vi "stop async modules.vi"(7 "Variant":variant, 8 "error in":errorcluster, 11 "Engine Data Out in":T1={"timed loop timer source"={"Processor"=0, "Priority"=0, "timing source dt"=0, "timer source"=refnum}, "control loop data"={"engine tag bus"={"Double"=[], "Single"=[], "I64"=[], "I32"=[], "I16"=[], "I8"=[], "U64"=[], "U32"=[], "U16"=[], "U8"=[], "Boolean"=[], "String"=[], "Array of Double"=[], "Array of Single"=[], "Array of I64"=[], "Array of I32"=[], "Array of I16"=[], "Array of I8"=[], "Array of U64"=[], "Array of U32"=[], "Array of U16"=[], "Array of U8"=[], "Array of Boolean"=[], "Array of String"=[]}, "engine schedule"={"module run flags"=[], "decimation schedule"={"decimations"=[], "offsets"=[]}}, "module information"=[]}, "status reporting"={"late? index (bool)"=0, "late count index (U32)"=0, "dt (ns) index (U64)"=0, "execution time (ns) index (U64)"=-1}}) -> (0 "error out":errorcluster, 3 "Engine Data Out out":T1={"timed loop timer source"={"Processor"=0, "Priority"=0, "timing source dt"=0, "timer source"=refnum}, "control loop data"={"engine tag bus"={"Double"=[], "Single"=[], "I64"=[], "I32"=[], "I16"=[], "I8"=[], "U64"=[], "U32"=[], "U16"=[], "U8"=[], "Boolean"=[], "String"=[], "Array of Double"=[], "Array of Single"=[], "Array of I64"=[], "Array of I32"=[], "Array of I16"=[], "Array of I8"=[], "Array of U64"=[], "Array of U32"=[], "Array of U16"=[], "Array of U8"=[], "Array of Boolean"=[], "Array of String"=[]}, "engine schedule"={"module run flags"=[], "decimation schedule"={"decimations"=[], "offsets"=[]}}, "module information"=[]}, "status reporting"={"late? index (bool)"=0, "late count index (U32)"=0, "dt (ns) index (U64)"=0, "execution time (ns) index (U64)"=-1}})   [LabVIEW 2013, in "main engine.lvlib"]
doc: "Requests that all asynchronous modules abort as quickly as possible. When the modules return we swap their data back into the main cluster so they can pretend they are synchronous modules for future operations."
uses:
  main engine.lvlib
  Engine Data.ctl
  <vilib>/NI/Module Timing Source/timing source/TBM timing source.lvclass
  timed loop timing sources.ctl
  control loop data.ctl
  <vilib>/NI/Tag Bus/table/data table.ctl
  engine run schedule.ctl
  engine decimation schedule.ctl
  full module data.ctl
  <vilib>/NI/Tag Bus Module Framework/runtime/TBM module execution interface.lvclass
  module run state.ctl
  async executor/asynchronous executor reference.ctl
  async executor/async message to executor.ctl
  Runtime/async command notification.ctl
  Runtime/async error info.ctl
  <vilib>/NI/Tag Bus Module Framework/runtime/error classification.ctl
  <vilib>/NI/Tag Bus Module Framework/module configuration/TBM module configuration.lvclass
  module method data.ctl
  <vilib>/NI/Tag Bus/table/transfer specification.ctl
  <vilib>/NI/Tag Bus/tag/Data Type.ctl
  fault handling spec.ctl
  Configuration/Error Actions.ctl
  status reporting data.ctl
  <vilib>/NI/Tag Bus/table/data table.lvlib
  <vilib>/NI/Tag Bus/tag/tag descriptor.lvclass
  Configuration/Standard Engine Configuration.lvclass
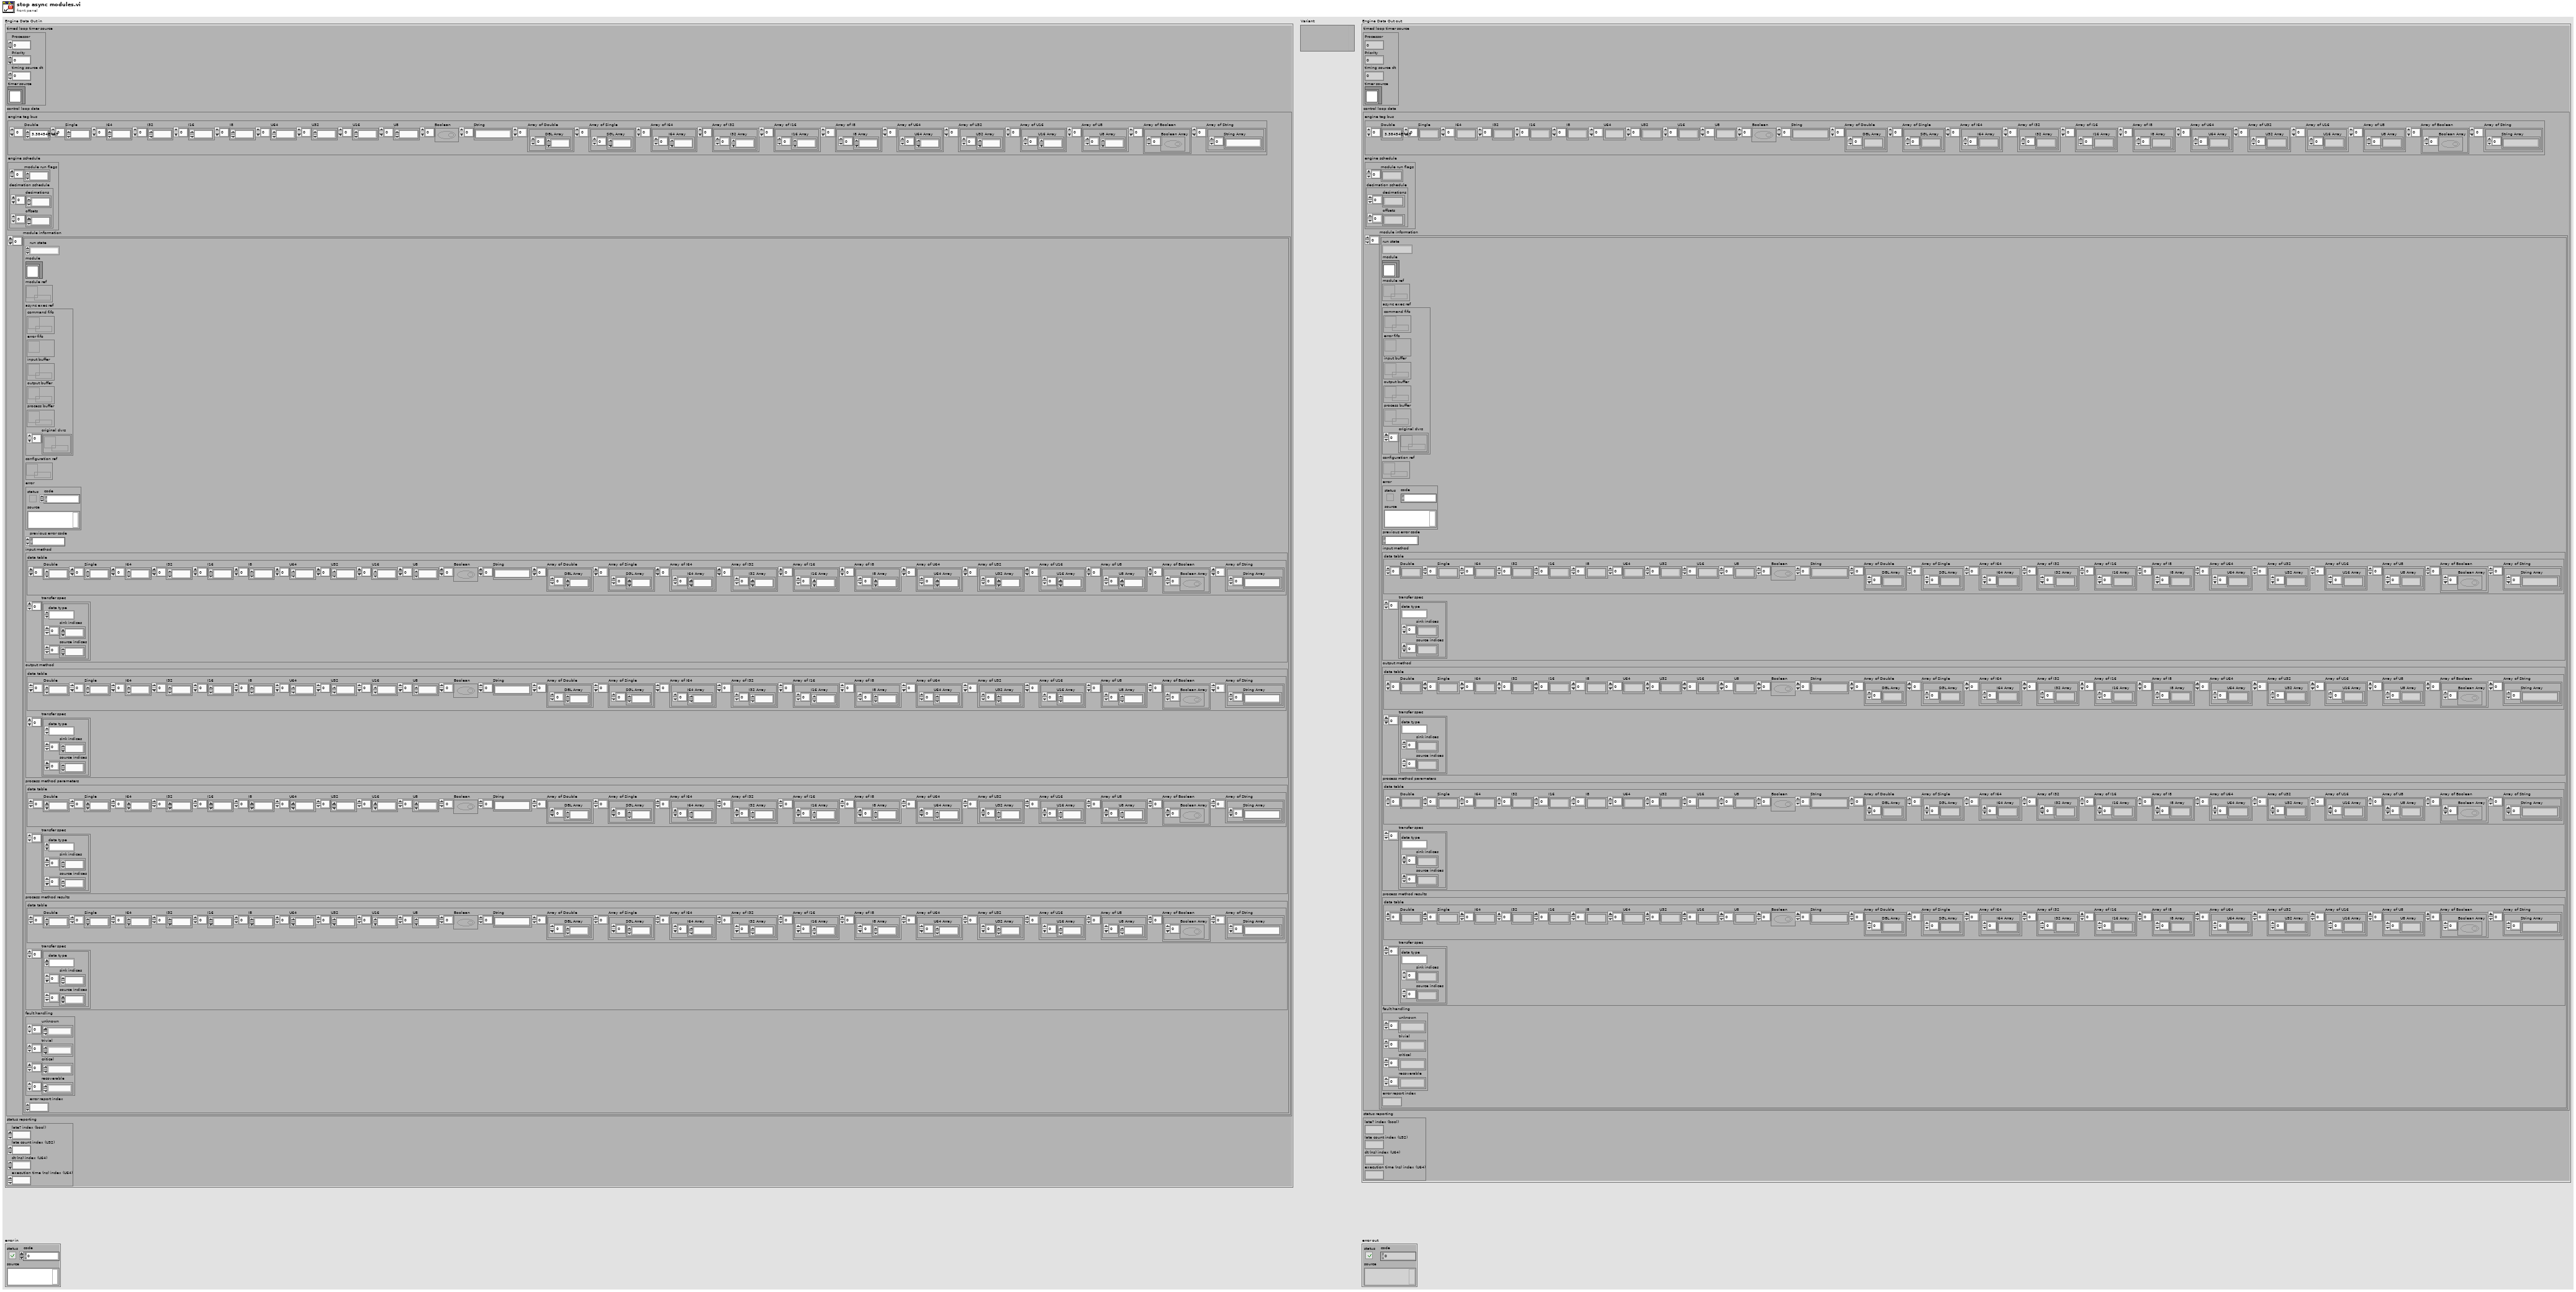
[diagram p1: front panel]
types:
  T1 = typedef "main engine.lvlib/Engine Data.ctl" = cluster{"timed loop timer source":T2, "control loop data":T3, "status reporting":T15}
  T2 = typedef "main engine.lvlib/timed loop timing sources.ctl" = cluster{"Processor":i32, "Priority":i32, "timing source dt":u32, "timer source":refnum<class "TBM timing source.lvclass">}
  T3 = typedef "main engine.lvlib/control loop data.ctl" = cluster{"engine tag bus":T4, "engine schedule":T5, "module information":T7[]}
  T4 = typedef "tag bus.lvlib/data table.lvlib/data table.ctl" = cluster{"Double":dbl[], "Single":sgl[], "I64":i64[], "I32":i32[], "I16":i16[], "I8":i8[], "U64":u64[], "U32":u32[], "U16":u16[], "U8":u8[], "Boolean":bool[], "String":string[], "Array of Double":cluster{"DBL Array":dbl[]}[], "Array of Single":cluster{"SGL Array":sgl[]}[], "Array of I64":cluster{"I64 Array":i64[]}[], "Array of I32":cluster{"I32 Array":i32[]}[], "Array of I16":cluster{"I16 Array":i16[]}[], "Array of I8":cluster{"I8 Array":i8[]}[], "Array of U64":cluster{"U64 Array":u64[]}[], "Array of U32":cluster{"U32 Array":u32[]}[], "Array of U16":cluster{"U16 Array":u16[]}[], "Array of U8":cluster{"U8 Array":u8[]}[], "Array of Boolean":cluster{"Boolean Array":bool[]}[], "Array of String":cluster{"String Array":string[]}[]}
  T5 = typedef "main engine.lvlib/engine run schedule.ctl" = cluster{"module run flags":u8[], "decimation schedule":T6}
  T6 = typedef "main engine.lvlib/engine decimation schedule.ctl" = cluster{"decimations":u16[], "offsets":u16[]}
  T7 = typedef "main engine.lvlib/full module data.ctl" = cluster{"run state":T8, "module":refnum<class "TBM module execution interface.lvclass">, "module ref":refnum<data-value>, "async exec ref":T9, "configuration ref":refnum<data-value>, "error":errorcluster, "previous error code":i32, "input method":T10, "output method":T10, "process method parameters":T10, "process method results":T10, "fault handling":T13, "error report index ":i32}
  T8 = typedef "main engine.lvlib/module run state.ctl" = enum16{"sync", "async"}
  T9 = typedef "main engine.lvlib/asynchronous executor reference.ctl" = cluster{"command fifo":refnum<k33>, "error fifo":refnum<k33>, "input buffer":refnum<k33>, "output buffer":refnum<k33>, "process buffer":refnum<k33>, "original dvrs":refnum<data-value>[]}
  T10 = typedef "main engine.lvlib/module method data.ctl" = cluster{"data table":T4, "transfer spec":T11[]}
  T11 = typedef "tag bus.lvlib/data table.lvlib/transfer specification.ctl" = cluster{"data type":T12, "sink indices":i32[], "source indices":i32[]}
  T12 = typedef "tag bus.lvlib/tag descriptor.lvclass/Data Type.ctl" = enum16{"Double", "Single", "I64", "I32", "I16", "I8", "U64", "U32", "U16", "U8", "Boolean", "String", "Array of Double", "Array of Single", "Array of I64", "Array of I32", "Array of I16", "Array of I8", "Array of U64", "Array of U32", "Array of U16", "Array of U8", "Array of Boolean", "Array of String"}
  T13 = typedef "main engine.lvlib/fault handling spec.ctl" = cluster{"unknown":T14[], "trivial":T14[], "critical":T14[], "recoverable":T14[]}
  T14 = typedef "Standard Engine Configuration.lvclass/Error Actions.ctl" = enum16{"Clear", "Notify", "Stop Component", "Stop Engine", "Safe State", "Attempt Recovery"}
  T15 = typedef "main engine.lvlib/status reporting data.ctl" = cluster{"late? index (bool)":i32, "late count index (U32)":i32, "dt (ns) index (U64)":i32, "execution time (ns) index (U64)":i32}
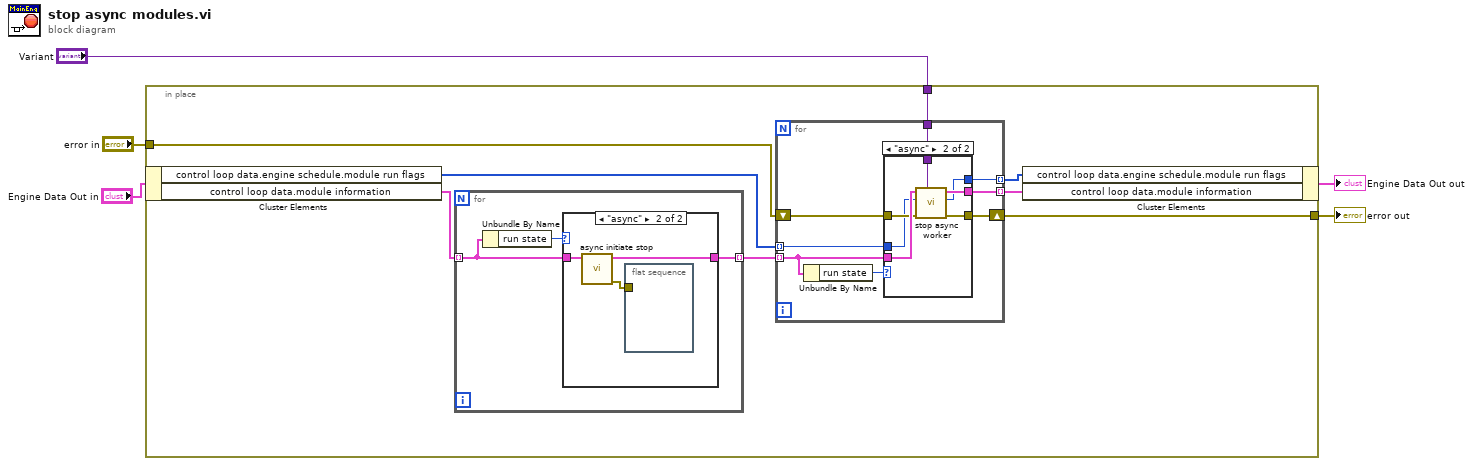
[diagram p0: block diagram]
diagram:
  n1 = in-place {
    in-place-border: "error in" -> [w10]
    in-place-border: [w9] -> w3
    in-place-border: "Variant" -> [w6]
    n2 = in-place-cluster #1("Engine Data Out in") -> ("control loop data.engine schedule.module run flags"=w11:u8[], "control loop data.module information"=w8:T7[])
    n3 = for {
      tunnel: w8 -> [w14] mode=indexing
      tunnel: [w15] -> w7 mode=indexing
      n4 = Unbundle By Name(w14) -> ("run state"=w16:T8)
      n5 = case shown="\"async\"" w16 {
        tunnel: [w17 w19] -> w15
        tunnel: w14 -> [w17 w20]
        frame "sync" {
        }
        frame "async" {
          n6 = call "async initiate stop.vi"("module data in"=w20) -> ("error out"=w18:errorcluster, "module data out"=w19:T7)  [unwired: 9 in]
          n7 = flat-sequence {
            tunnel: w18 -> [_]
            frame #0 {
            }
          }
        }
      }
    }
    n8 = for {
      tunnel: w7 -> [w26] mode=indexing
      tunnel: [w27] -> w13 mode=indexing
      tunnel: [w25] -> w12 mode=indexing
      tunnel: w11 -> [w24] mode=indexing
      shift-right: [w23] -> w9
      shift-left: w10 -> [w22]
      tunnel: w6 -> [w21]
      n9 = Unbundle By Name(w26) -> ("run state"=w28:T8)
      n10 = case shown="\"async\"" w28 {
        tunnel: [w31 w35] -> w27
        tunnel: w26 -> [w31 w38]
        tunnel: [w30 w33] -> w25
        tunnel: w24 -> [w30 w34]
        tunnel: [w29 w36] -> w23
        tunnel: w22 -> [w29 w37]
        tunnel: w21 -> [_ w32]
        frame "sync" {
        }
        frame "async" {
          n11 = call "stop async worker.vi"("Variant"=w32, "error in"=w37, "run flag in"=w34, "module data in"=w38) -> ("error out"=w36:errorcluster, "run flag out"=w33:u8, "module data out"=w35:T7)  [unwired: 5 in]
        }
      }
    }
    n12 = in-place-cluster #1("control loop data.engine schedule.module run flags"=w12, "control loop data.module information"=w13) -> (→"Engine Data Out out":T1)
  }
  "error out" <- w3
